vi "Select Index.vi"(3 "Indexes":i32[](array[numeric]), 4 "Array In":cluster{"x":sgl, "y":sgl}[](array[cluster]), 5 "Function In":cluster{"Z":dbl[], "Score":sgl[]}) -> (1 "Array Out":cluster{"x":sgl, "y":sgl}[](array[cluster]), 2 "Function Out":cluster{"Z":dbl[], "Score":sgl[]})   [LabVIEW 2014]
panel:
  # "LICENSED MATERIALS – PROPERTY OF IBM\nCopyright IBM Corp. 2016,\nALL RIGHTS RESERVED"
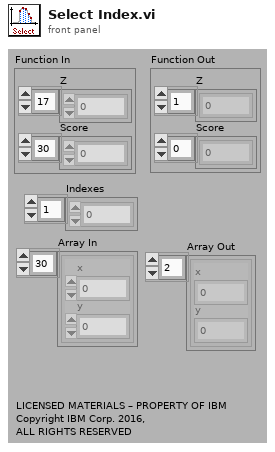
[diagram p1: front panel]
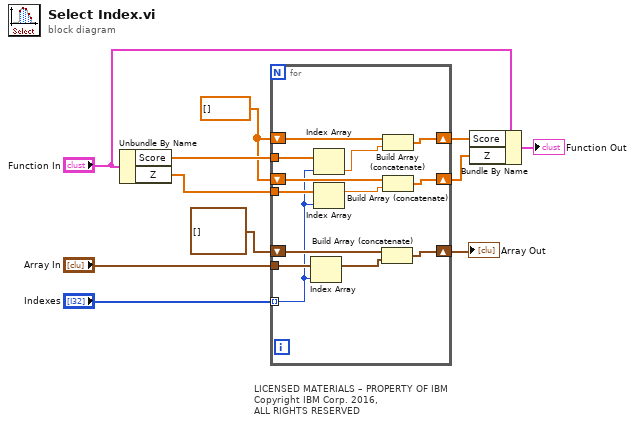
[diagram p0: block diagram]
diagram:
  w7 = dbl[] [] ("Array")
  # "LICENSED MATERIALS – PROPERTY OF IBM\nCopyright IBM Corp. 2016,\nALL RIGHTS RESERVED"
  n1 = Unbundle By Name("Function In") -> ("Score"=w9:sgl[], "Z"=w8:dbl[])
  n2 = for {
    tunnel: w9 -> [w19]
    shift-right: [w23] -> w6
    shift-left: w7 -> [w24]
    tunnel: w8 -> [w20]
    shift-right: [w22] -> w5
    shift-left: w7 -> [w21]
    tunnel: "Indexes" -> [w13] mode=indexing
    tunnel: "Array In" -> [w18]
    shift-right: [w12] -> w1
    shift-left: cluster{"x":sgl, "y":sgl}[] [] ("Array In 2") -> [w17]
    n3 = Index Array(array=w18, index=w13) -> (element=w14:cluster{"x":sgl, "y":sgl})
    n4 = Index Array(array=w19, index=w13) -> (element=w15:sgl)
    n5 = Index Array(array=w20, index=w13) -> (element=w16:dbl)
    n6 = Build Array (concatenate)(w17, w14) -> (w12:cluster{"x":sgl, "y":sgl}[])
    n7 = Build Array (concatenate)(w24, w15) -> (w23:dbl[])
    n8 = Build Array (concatenate)(w21, w16) -> (w22:dbl[])
  }
  "Array Out" <- w1
  n9 = Bundle By Name(cluster="Function In", "Score"=w6, "Z"=w5) -> (→"Function Out":cluster{"Z":dbl[], "Score":sgl[]})
